vi "AutoMatchBrianSheridan.vi"() -> ()   [LabVIEW 2014]
panel:
  out "# of iterations":dbl format="%#.0f"
  out "Current Number":dbl format="%#.0f"
  in  "Number to Match":dbl min=0.0 max=1000.0 step=1.0 format="%#.0f"
  # "*number indicator*"
  # "*numeric control*"
  # "Precision = 0"
  # "Data Range"
  # "Default = 50"
  # "Min = 0 (Coerce)"
  # "Max = 1000 (Coerce)"
  # "Inc = 1 ( Coerce to Nearest)"
  # "*number indicator*"
  # "Precision = 0"
  # "Precision = 0"
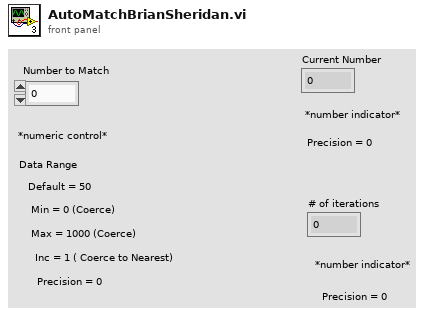
[diagram p1: front panel]
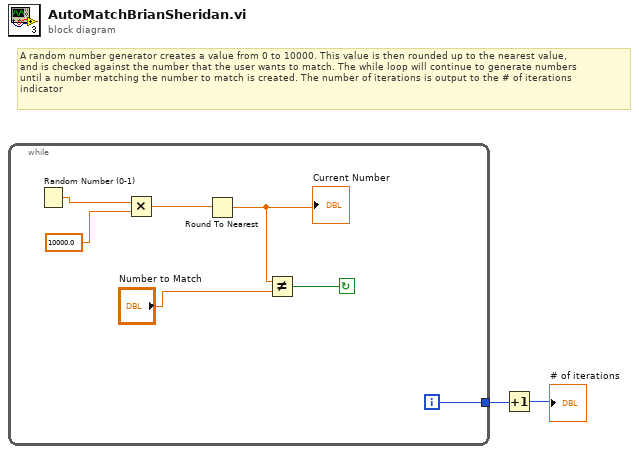
[diagram p0: block diagram]
diagram:
  # "A random number generator creates a value from 0 to 10000. This value is then rounded up to the nearest value,\nand is checked against the number that the user wants to match. The while loop will continue to generate numbers \nuntil a number matching the number to match is created. The number of iterations is output to the # of iterations \nindicator"
  n1 = while {
    tunnel: [w3] -> w2
    i -> [w3]
    stop <- w6 continue-if-true
    n2 = Random Number (0-1)() -> (number: 0 to 1=w9:dbl)
    n3 = Multiply(x=w9, y=10000.0) -> (x*y=w7:dbl)
    n4 = Round To Nearest(number=w7) -> (nearest integer value=w4:dbl)
    "Current Number" <- w4
    n5 = Not Equal?(x=w4, y="Number to Match") -> (x != y?=w6:bool)
  }
  n6 = Increment(x=w2) -> (x+1=→"# of iterations":i32)
